vi "Convert RAWDATA.vi"(0 "VIS-IR in":refnum<class "VIS-IR.lvclass">, 1 "# of scan":i32, 2 "WCM_limits":T1, 3 "I channel seq IN":cluster{"BG":i32[], "Ie":i32[], "I0":i32[]}[](array[cluster]), 5 "I channel":i32[][](array[numeric]), 7 "WCM_values IN":sgl[](array[numeric]), 9 "II channel":i32[][](array[numeric]), 11 "error in (no error)":errorcluster, 12 "All?":bool=TRUE, 13 "WCM_corrections":bool, 14 "II channel seq IN":cluster{"BG":i32[], "Ie":i32[], "I0":i32[]}[](array[cluster])) -> (4 "VIS-IR out":refnum<class "VIS-IR.lvclass">, 6 "I channel seq":cluster{"BG":i32[], "Ie":i32[], "I0":i32[]}[](array[cluster]), 8 "WCM_values OUT":sgl[](array[numeric]), 10 "II channel seq":cluster{"BG":i32[], "Ie":i32[], "I0":i32[]}[](array[cluster]), 15 "error out":errorcluster)   [LabVIEW 2015, in "VIS-IR.lvclass"]
uses:
  VIS-IR.lvclass
  dependecies/ControlsVIs/Clusters-def/Def_WCM_limits.ctl
  Detector.lvclass
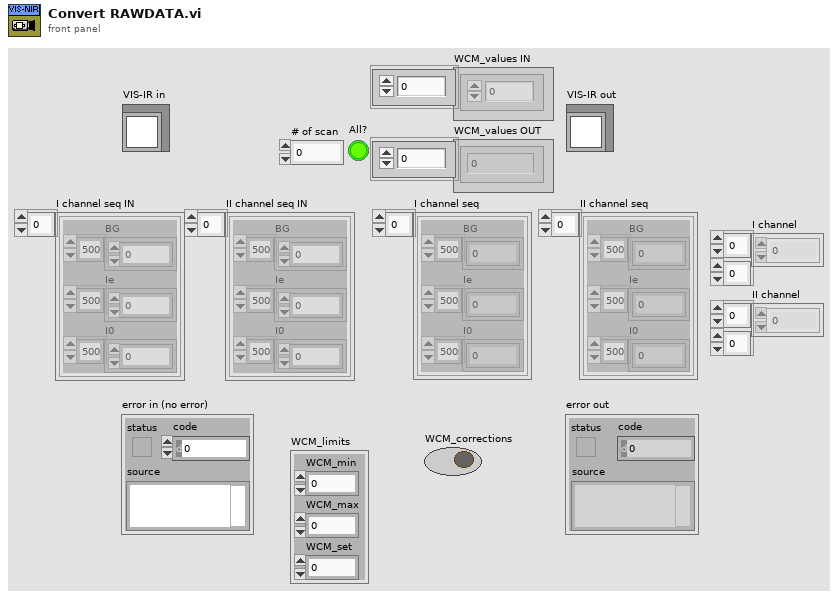
[diagram p1: front panel]
types:
  T1 = typedef "Def_WCM_limits.ctl" = cluster{"WCM_min":dbl, "WCM_max":dbl, "WCM_set":dbl}
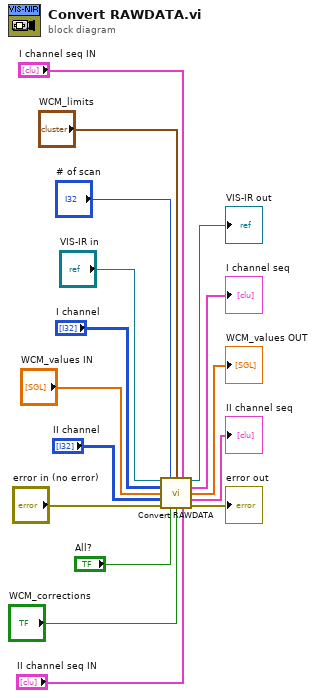
[diagram p0: block diagram]
diagram:
  n1 = call-parent "Convert RAWDATA.vi"("Detector in"="VIS-IR in", "# of scan"="# of scan", "WCM_limits"="WCM_limits", "I channel seq IN"="I channel seq IN", "I channel"="I channel", "WCM_values IN"="WCM_values IN", "II channel"="II channel", "error in (no error)"="error in (no error)", "All?"="All?", "WCM_corrections"="WCM_corrections", "II channel seq IN"="II channel seq IN") -> ("Detector out"=→"VIS-IR out":refnum<class "VIS-IR.lvclass">, "I channel seq"=→"I channel seq":cluster{"BG":i32[], "Ie":i32[], "I0":i32[]}[], "WCM_values OUT"=→"WCM_values OUT":sgl[], "II channel seq"=→"II channel seq":cluster{"BG":i32[], "Ie":i32[], "I0":i32[]}[], "error out"=→"error out":errorcluster)
